vi "UpdateCriteriaResult.vi"(10 "Data ain":string, 11 "Criteria In":string) -> (0 "Error Out":errorcluster, 2 "PASS?":string, 3 "Criteria":string)   [LabVIEW 2019]
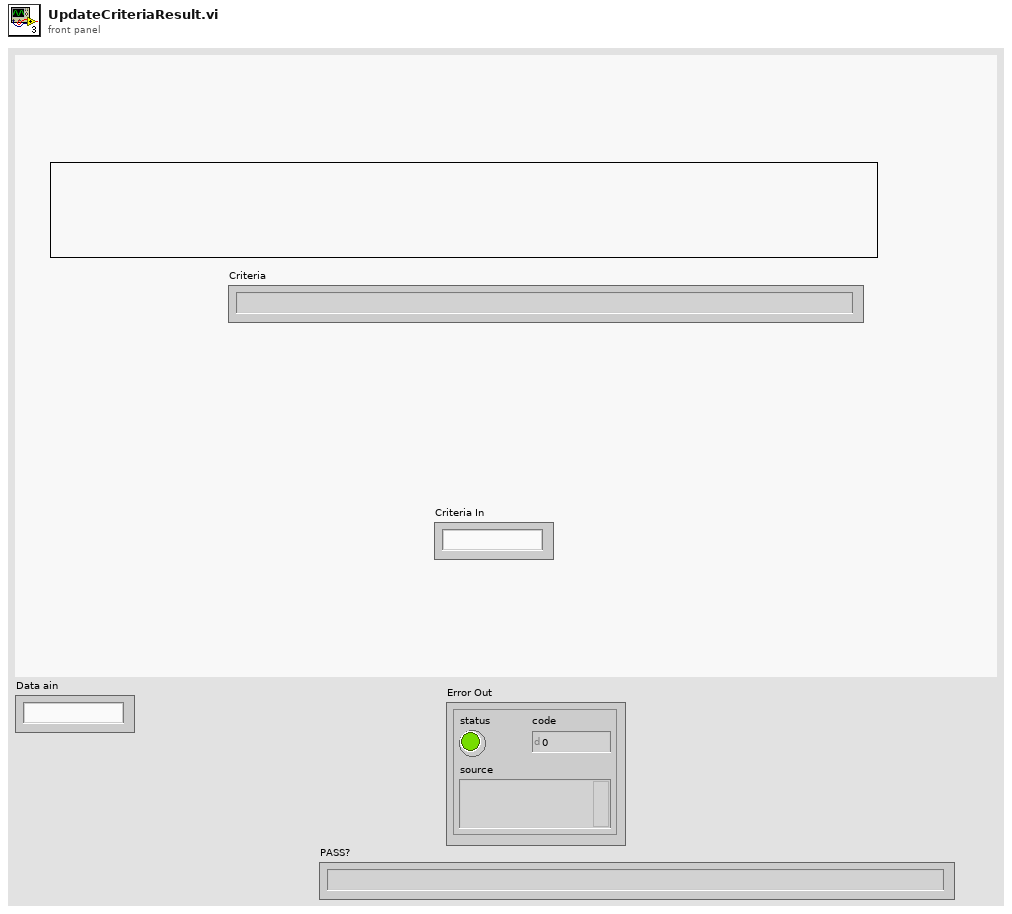
[diagram p1: front panel]
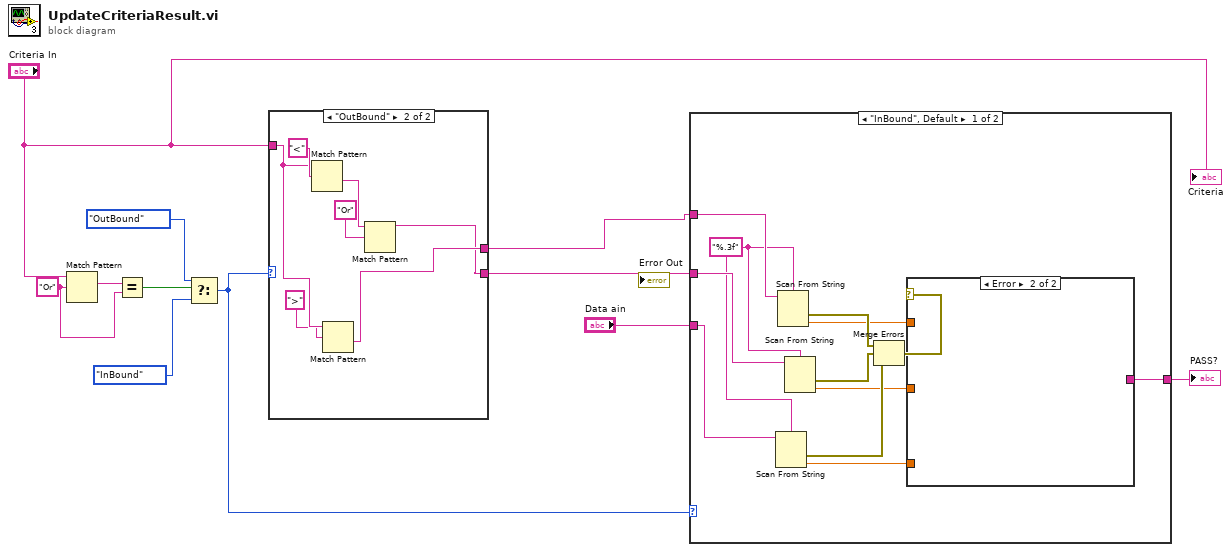
[diagram p0: block diagram]
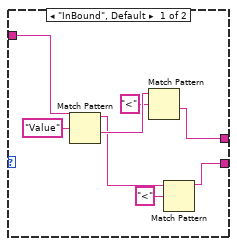
[diagram p2: hidden frame]
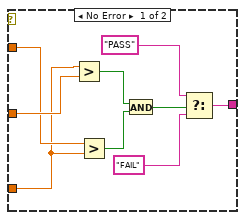
[diagram p3: hidden frame]
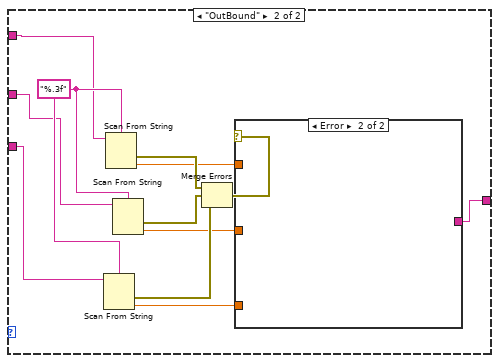
[diagram p4: hidden frame]
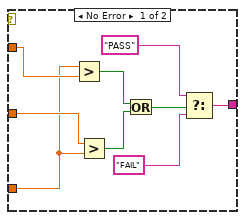
[diagram p5: hidden frame]
diagram:
  w9 = "Or" ("regular expression")
  n1 = Match Pattern(string="Criteria In", regular expression=w9) -> (match substring=w10:string)  [unwired: 1 in, 3 out]
  n2 = Equal?(x=w10, y=w9) -> (x = y?=w8:bool)
  n3 = Select(t=enum16{"InBound", "OutBound"}."OutBound" ("Condition"), s=w8, f=enum16{"InBound", "OutBound"}."InBound" ("Condition")) -> (s? t:f=w4:enum16{"InBound", "OutBound"})
  n4 = case shown="\"OutBound\"" w4 {
    tunnel: "Criteria In" -> [w19 w23]
    tunnel: [w12 w20] -> w3
    tunnel: [w15 w21] -> w2
    frame "InBound", Default {
      n5 = Match Pattern(string=w19, regular expression="Value") -> (before substring=w14:string, after substring=w17:string)  [unwired: 1 in, 2 out]
      n6 = Match Pattern(string=w17, regular expression="<") -> (after substring=w15:string)  [unwired: 1 in, 3 out]
      n7 = Match Pattern(string=w14, regular expression="<") -> (before substring=w12:string)  [unwired: 1 in, 3 out]
    }
    frame "OutBound" {
      n8 = Match Pattern(string=w23, regular expression="<") -> (after substring=w24:string)  [unwired: 1 in, 3 out]
      n9 = Match Pattern(string=w23, regular expression=">") -> (after substring=w21:string)  [unwired: 1 in, 3 out]
      n10 = Match Pattern(string=w24, regular expression="Or") -> (before substring=w20:string)  [unwired: 1 in, 3 out]
    }
  }
  n11 = case shown="\"InBound\", Default" w4 {
    tunnel: w3 -> [w38 w50]
    tunnel: w2 -> [w36 w51]
    tunnel: "Data ain" -> [w37 w49]
    tunnel: [w27 w48] -> w11
    frame "InBound", Default {
      w35 = "%.3f" ("format string")
      n12 = Scan From String(format string=w35, input string=w37) -> (error out=w32:errorcluster, output 1=w30:dbl)  [unwired: 3 in, 2 out]
      n13 = Scan From String(format string=w35, input string=w36) -> (error out=w34:errorcluster, output 1=w28:dbl)  [unwired: 3 in, 2 out]
      n14 = Scan From String(format string=w35, input string=w38) -> (error out=w33:errorcluster, output 1=w29:dbl)  [unwired: 3 in, 2 out]
      n15 = Merge Errors(w34, w33, w32) -> (w31:errorcluster)
      n16 = case shown="Error" w31 {
        tunnel: w30 -> [w45 _]
        tunnel: w29 -> [w47 _]
        tunnel: w28 -> [w46 _]
        tunnel: [w39 _] -> w27
        frame No Error {
          n17 = Greater?(x=w45, y=w47) -> (0:w44:bool)
          n18 = Greater?(x=w46, y=w45) -> (0:w43:bool)
          n19 = And(x=w44, y=w43) -> (x .and. y?=w42:bool)
          n20 = Select(t="PASS" ("string"), s=w42, f="FAIL" ("string")) -> (s? t:f=w39:string)
        }
        frame Error {
        }
      }
    }
    frame "OutBound" {
      w59 = "%.3f" ("format string")
      n21 = Scan From String(format string=w59, input string=w49) -> (error out=w56:errorcluster, output 1=w54:dbl)  [unwired: 3 in, 2 out]
      n22 = Scan From String(format string=w59, input string=w51) -> (error out=w58:errorcluster, output 1=w52:dbl)  [unwired: 3 in, 2 out]
      n23 = Scan From String(format string=w59, input string=w50) -> (error out=w57:errorcluster, output 1=w53:dbl)  [unwired: 3 in, 2 out]
      n24 = Merge Errors(w58, w57, w56) -> (w55:errorcluster)
      n25 = case shown="Error" w55 {
        tunnel: w54 -> [w60 _]
        tunnel: w53 -> [w61 _]
        tunnel: w52 -> [w62 _]
        tunnel: [w63 _] -> w48
        frame No Error {
          n26 = Greater?(x=w60, y=w62) -> (0:w68:bool)
          n27 = Greater?(x=w61, y=w60) -> (0:w67:bool)
          n28 = Or(x=w68, y=w67) -> (x .or. y?=w66:bool)
          n29 = Select(t="PASS" ("string"), s=w66, f="FAIL" ("string")) -> (s? t:f=w63:string)
        }
        frame Error {
        }
      }
    }
  }
  "PASS?" <- w11
  "Criteria" <- "Criteria In"
